vi "ReadEncoderDirection.vi"(8 "error in":errorcluster, 9 "IP address":string, 10 "Axis":enum16{"Z", "Y", "X"}(ring), 11 "connection refnum in":refnum<k5>) -> (0 "error out":errorcluster, 1 "Boolean Array":bool[](array[boolean]), 2 "Encoder Direction":string, 3 "connection refnum out":refnum<k5>)   [LabVIEW 2023]
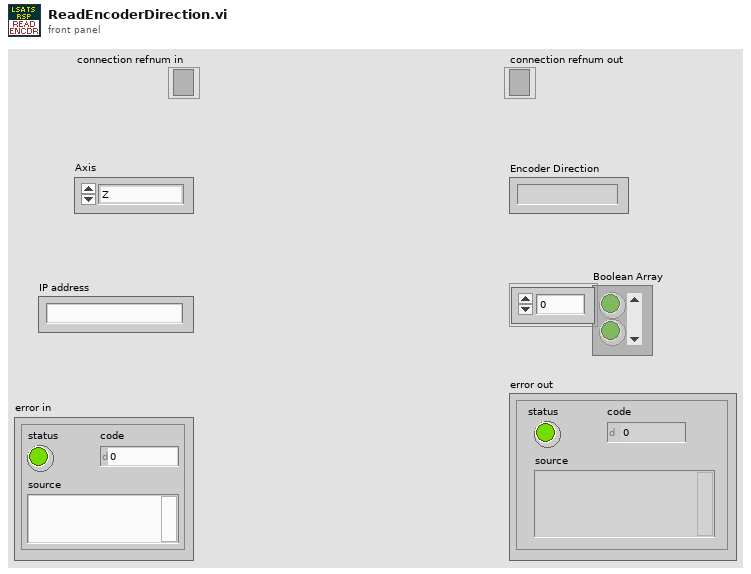
[diagram p1: front panel]
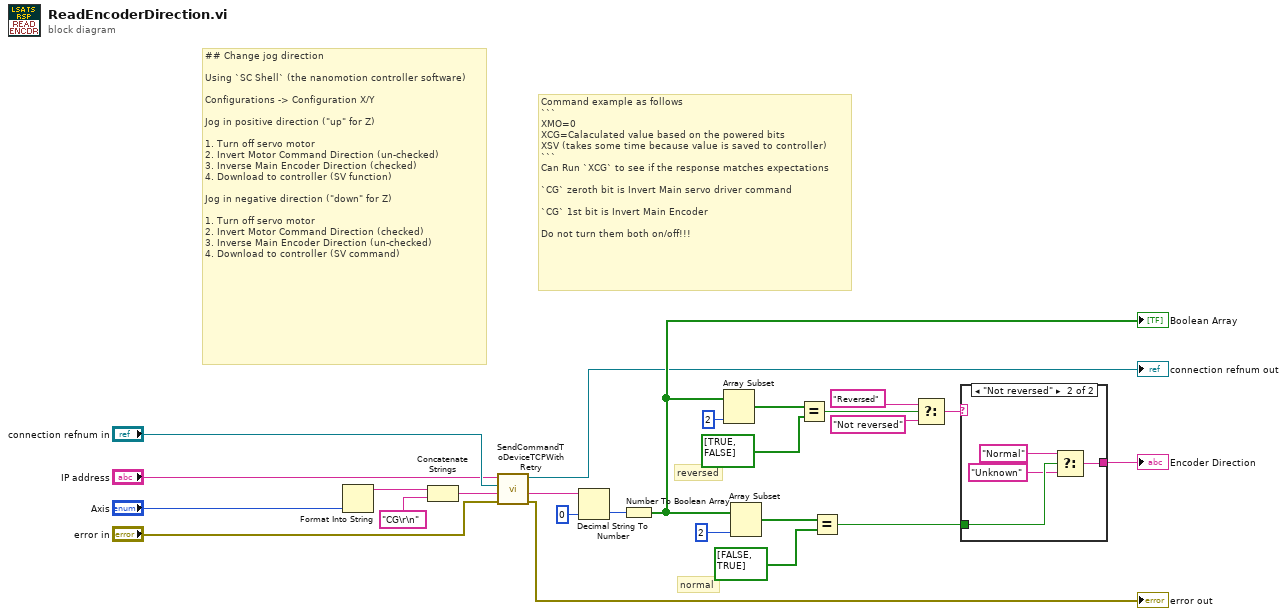
[diagram p0: block diagram]
diagram:
  # "normal"
  # "reversed"
  # "Command example as follows\n```\nXMO=0\nXCG=Calaculated value based on the powered bits\nXSV (takes some time because value is saved to controller)\n```\nCan Run `XCG` to see if the response matches expectations\n\n`CG` zeroth bit is Invert Main servo driver command\n\n`CG` 1st bit is Invert Main Encoder\n\nDo not turn them both on/off!!!"
  # "## Change jog direction\n\nUsing `SC Shell` (the nanomotion controller software)\n\nConfigurations -> Configuration X/Y\n\nJog in positive direction (\"up\" for Z)\n\n1. Turn off servo motor\n2. Invert Motor Command Direction (un-checked)\n3. Inverse Main Encoder Direction (checked)\n4. Download to controller (SV function)\n\nJog in negative direction (\"down\" for Z)\n\n1. Turn off servo motor\n2. Invert Motor Command Direction (checked)\n3. Inverse Main Encoder Direction (un-checked)\n4. Download to controller (SV command)"
  n1 = Format Into String("Axis") -> (resulting string=w20:string)  [unwired: 3 in, 1 out]
  n2 = Concatenate Strings(w20, "CG\r\n" ("string")) -> (w24:string)
  n3 = call "SendCommandToDeviceTCPWithRetry.vi"("error in"="error in", "str command"=w24, "connection refnum in"="connection refnum in", "IP address"="IP address") -> ("error out"=→"error out":errorcluster, "str out"=w23:string, "connection refnum out"=→"connection refnum out":refnum<k5>)  [unwired: 4 in, 1 out]
  n4 = Decimal String To Number(string=w23, default (0L)=u16 0 ("original number 2")) -> (number=w21:u16)  [unwired: 1 in, 1 out]
  n5 = Number To Boolean Array(number=w21) -> (Boolean array=w8:bool[])
  "Boolean Array" <- w8
  n6 = Array Subset(array=w8, length=2) -> (w16:bool[])  [unwired: 1 in]
  n7 = Array Subset(array=w8, length=2) -> (w7:bool[])  [unwired: 1 in]
  n8 = Equal?(x=w16, y=bool[] [TRUE, FALSE]) -> (x = y?=w13:bool)
  n9 = Equal?(x=w7, y=bool[] [FALSE, TRUE]) -> (x = y?=w10:bool)
  n10 = Select(t="Reversed", s=w13, f="Not reversed") -> (s? t:f=w11:string)
  n11 = case shown="\"Not reversed\"" w11 {
    selector: w11 -> [w26 _]
    tunnel: w10 -> [_ w30]
    tunnel: [w26 w27] -> w9
    frame "Reversed", Default {
    }
    frame "Not reversed" {
      n12 = Select(t="Normal", s=w30, f="Unknown") -> (s? t:f=w27:string)
    }
  }
  "Encoder Direction" <- w9
